vi "4Pi Dual DM - No Zeros Mean.vi"(7 "Image IN":dbl[][](array[numeric]), 13 "STDev Factor":dbl format="%#_13g") -> (8 "No Zero Mean":dbl format="%0.2f")   [LabVIEW 2016]
uses:
  <vilib>/Analysis/baseanly.llb/Mean (DBL).vi
  <vilib>/Analysis/NI_AALBase.lvlib
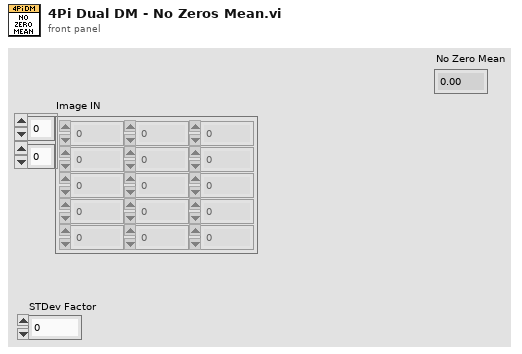
[diagram p1: front panel]
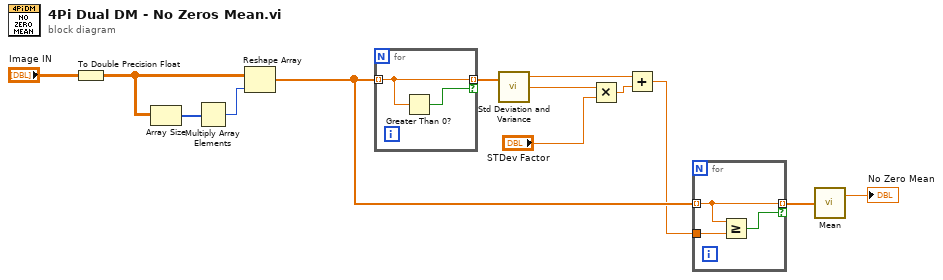
[diagram p0: block diagram]
diagram:
  n1 = To Double Precision Float(number="Image IN") -> (double precision float=w6:dbl[][])
  n2 = Array Size(array=w6) -> (size(s)=w13:i32[])
  n3 = Multiply Array Elements(1:w13) -> (0:w12:i32)
  n4 = Reshape Array(w6, w12) -> (w5:dbl[])
  n5 = for {
    tunnel: w5 -> [w15] mode=indexing
    tunnel: [w15] -> w2 mode=indexing if=w14
    n6 = Greater Than 0?(x=w15) -> (x > 0?=w14:bool)
  }
  n7 = call <vilib>:"Std Deviation and Variance.vi"("X"=w2) -> ("mean"=w8:dbl, "standard deviation"=w10:dbl)  [unwired: 1 in, 1 out]
  n8 = Multiply(x=w10, y="STDev Factor") -> (x*y=w7:dbl)
  n9 = Add(x=w8, y=w7) -> (x+y=w4:dbl)
  n10 = for {
    tunnel: w5 -> [w17] mode=indexing
    tunnel: w4 -> [w18]
    tunnel: [w17] -> w1 mode=indexing if=w16
    n11 = Greater Or Equal?(x=w17, y=w18) -> (x >= y?=w16:bool)
  }
  n12 = call-poly <vilib>:"Mean.vi"("X"=w1) -> ("mean"=→"No Zero Mean":dbl)  [unwired: 1 out]
